vi "motor_with_lidar_imitator.vi"() -> ()   [LabVIEW 2014]
uses:
  <vilib>/Instr/_visa.llb/VISA Configure Serial Port (Instr).vi
  <vilib>/Utility/file.llb/Write To Spreadsheet File (DBL).vi
panel:
  out "Angle":dbl
  out "Real iteration angle":dbl
  in  "Stop":bool
  in  "error in (no error)":errorcluster
  in  "Stop":dbl
  in  "Vertical resolution":dbl
  in  "VISA resource name":refnum<visa-resource-name>
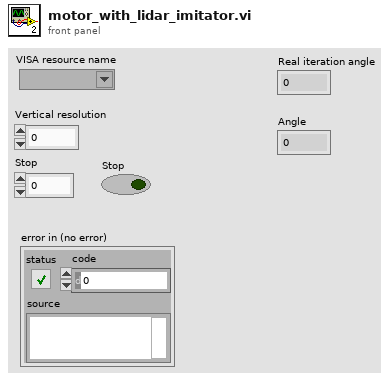
[diagram p1: front panel]
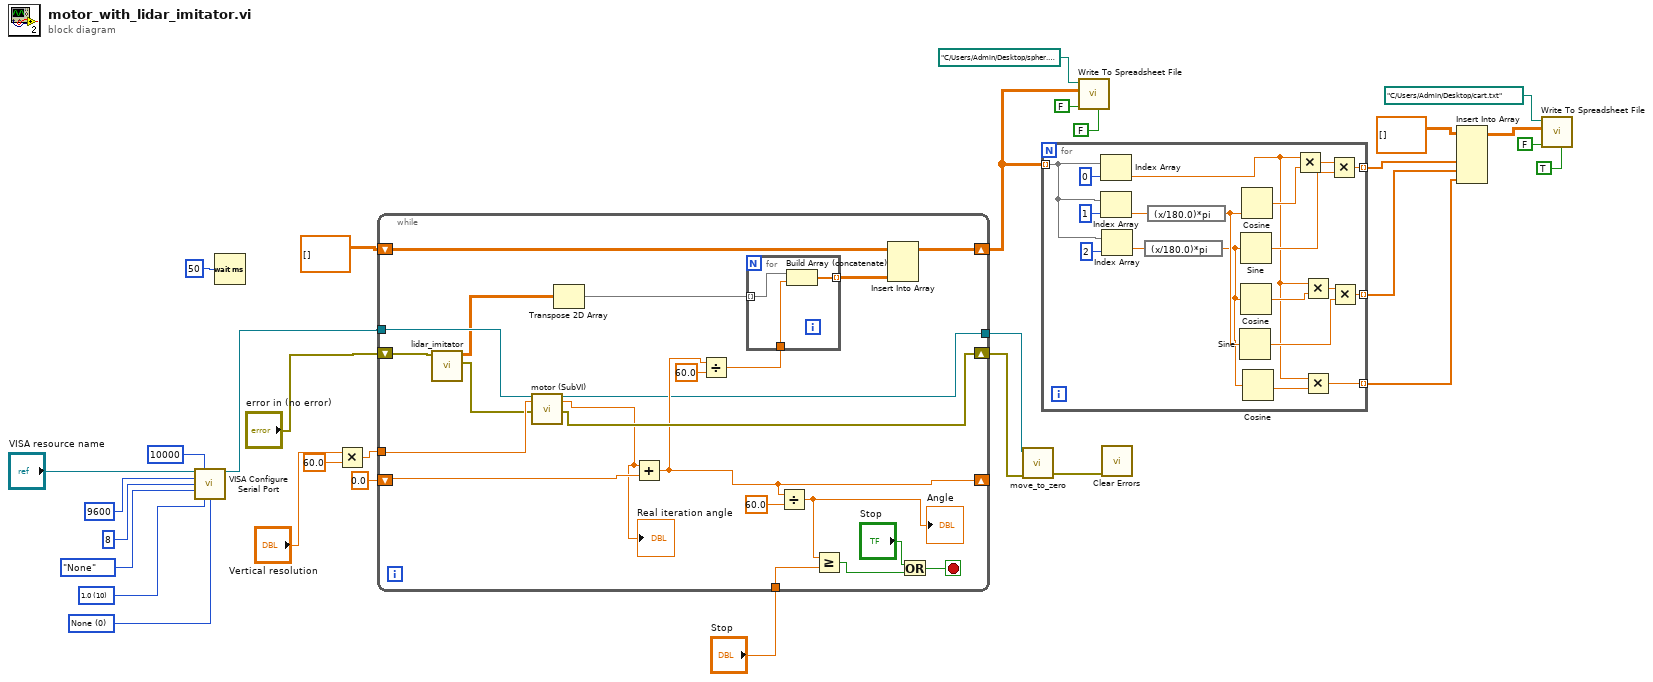
[diagram p0: block diagram]
diagram:
  w24 = u16 0 items=["None", "XON/XOFF", "RTS/CTS", "XON/XOFF & RTS/CTS", "DTR/DSR", "XON/XOFF & DTR/DSR"] ("flow control (0:none)")
  w25 = u16 10 items=["1.0"=10, "1.5"=15, "2.0"=20] ("stop bits (10: 1 bit)")
  n1 = call-poly "VISA Configure Serial Port"("VISA resource name"="VISA resource name", "timeout (10sec)"=u32 10000, "baud rate (9600)"=u32 9600, "data bits (8)"=u16 8, "parity (0:none)"=enum16{"None", "Odd", "Even", "Mark", "Space"}."None", "stop bits (10: 1 bit)"=w25, "flow control (0:none)"=w24) -> ("VISA resource name out"=w11:refnum<visa-resource-name>)  [unwired: 7 in, 1 out]
  n2 = Wait (ms)(milliseconds to wait=u32 50) -> ()  [unwired: 1 out]
  n3 = Multiply(x="Vertical resolution", y=60.0) -> (x*y=w22:dbl)
  n4 = while {
    tunnel: w11 -> [w52]
    tunnel: w22 -> [w53]
    shift-right: [w51] -> w12
    shift-left: "error in (no error)" -> [w50]
    tunnel: "Stop" -> [w43]
    shift-right: [w40] -> _
    shift-left: 0.0 -> [w45]
    shift-right: [w35] -> w6
    shift-left: dbl[][] [] -> [w36]
    tunnel: [w32] -> w14
    stop <- w46 stop-if-true
    n5 = call "lidar_imitator.vi"("error in (no error)"=w50) -> ("error out"=w49:errorcluster, "array"=w38:dbl[][])  [unwired: 9 in]
    n6 = call "motor (SubVI).vi"("VISA Refnum in"=w52, "step"=w53, "error in (no error)"=w49) -> ("VISA resource name out"=w32:refnum<visa-resource-name>, "Angle"=w33:dbl, "error out"=w51:errorcluster)  [unwired: 14 in]
    "Real iteration angle" <- w33
    n7 = Transpose 2D Array(2D array=w38) -> (transposed array=w37:dbl[][])
    n8 = Add(x=w33, y=w45) -> (x+y=w40:dbl)
    n9 = Divide(x=w40, y=60.0) -> (x/y=w39:dbl)
    n10 = for {
      tunnel: w37 -> [w54] mode=indexing
      tunnel: [w56] -> w34 mode=indexing
      tunnel: w39 -> [w55]
      n11 = Build Array (concatenate)(w54, w55) -> (w56:dbl[])
    }
    n12 = Divide(x=w40, y=60.0) -> (x/y=w42:dbl)
    "Angle" <- w42
    n13 = Greater Or Equal?(x=w42, y=w43) -> (x >= y?=w48:bool)
    n14 = Insert Into Array(array=w36, new element=w34) -> (w35:dbl[][])  [unwired: 2 in]
    n15 = Or(x="Stop", y=w48) -> (x .or. y?=w46:bool)
  }
  n16 = call "move_to_zero.vi"("error in (no error)"=w12, "VISA Refnum in"=w14) -> ("error out"=w13:errorcluster)  [unwired: 8 in, 1 out]
  n17 = for {
    tunnel: w6 -> [w72] mode=indexing
    tunnel: [w68] -> w4 mode=indexing
    tunnel: [w61] -> w2 mode=indexing
    tunnel: [w57] -> w1 mode=indexing
    n18 = Index Array(array=w72, index=0) -> (element=w59:dbl)
    n19 = Index Array(array=w72, index=1) -> (element=w66:dbl)
    n20 = Index Array(array=w72, index=2) -> (element=w67:dbl)
    n21 = expression code="(x/180.0)*pi"(w67) -> (w60:dbl)
    n22 = expression code="(x/180.0)*pi"(w66) -> (w65:dbl)
    n23 = Sine(x=w65) -> (sin(x)=w62:dbl)
    n24 = Sine(x=w60) -> (sin(x)=w69:dbl)
    n25 = Cosine(x=w60) -> (cos(x)=w64:dbl)
    n26 = Cosine(x=w65) -> (cos(x)=w71:dbl)
    n27 = Cosine(x=w60) -> (cos(x)=w58:dbl)
    n28 = Multiply(x=w59, y=w71) -> (x*y=w70:dbl)
    n29 = Multiply(x=w59, y=w64) -> (x*y=w63:dbl)
    n30 = Multiply(x=w59, y=w58) -> (x*y=w57:dbl)
    n31 = Multiply(x=w70, y=w69) -> (x*y=w68:dbl)
    n32 = Multiply(x=w63, y=w62) -> (x*y=w61:dbl)
  }
  n33 = call-poly <vilib>:"Write To Spreadsheet File.vi"("transpose? (no:F)"=FALSE, "append to file? (new file:F)"=FALSE, "2D data"=w6, "file path (dialog if empty)"=path "C:/Users/Admin/Desktop/spher.txt") -> ()  [unwired: 4 in, 1 out]
  n34 = call <vilib>:"Clear Errors.vi"("error in (no error)"=w13) -> ()  [unwired: 5 in, 2 out]
  n35 = Insert Into Array(array=dbl[][] [], new element #1=w4, new element #2=w2, new element #3=w1) -> (w3:dbl[][])  [unwired: 2 in]
  n36 = call-poly <vilib>:"Write To Spreadsheet File.vi"("transpose? (no:F)"=TRUE, "append to file? (new file:F)"=FALSE, "2D data"=w3, "file path (dialog if empty)"=path "C:/Users/Admin/Desktop/cart.txt") -> ()  [unwired: 4 in, 1 out]
